vi "newDDreference.vi"(0 "Engine Reference":refnum<k7>, 5 "Sequence File Ref":refnum<k7>, 11 "error in":errorcluster) -> (4 "Engine Reference (out)":refnum<k7>, 6 "Sequence File (out)":refnum<k7>, 15 "error out":errorcluster)   [LabVIEW 2010]
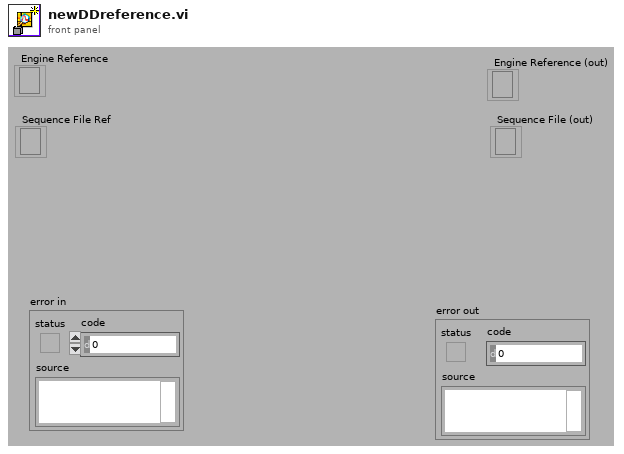
[diagram p1: front panel]
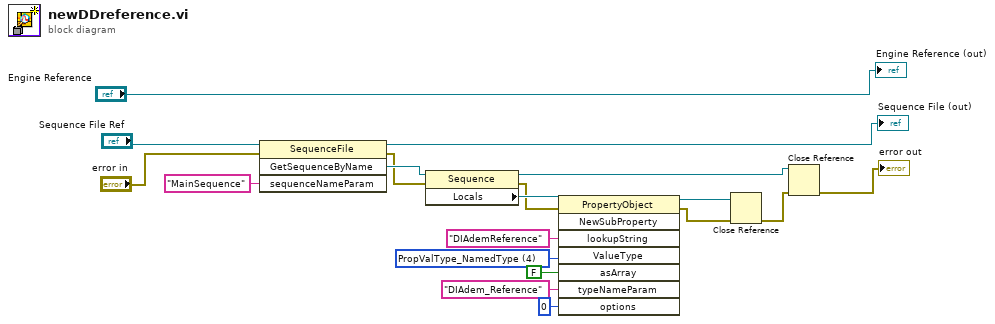
[diagram p0: block diagram]
diagram:
  w15 = 4 items=["PropValType_Container", "PropValType_String", "PropValType_Boolean", "PropValType_Number", "PropValType_NamedType", "PropValType_Reference", "PropValType_Array"] ("ValueType")
  n1 = invoke class="SequenceFile" method="GetSequenceByName"(reference="Sequence File Ref", error in="error in", "sequenceNameParam"="MainSequence") -> (reference out=→"Sequence File (out)":refnum<k7>, error out=w1:errorcluster, "GetSequenceByName"=w18:refnum<k7>)  [unwired: 1 in, 1 out]
  n2 = property class="Sequence"(reference=w18, error in=w1) -> (reference out=w7:refnum<k7>, error out=w9:errorcluster, "Locals"=w17:refnum<k7>)
  n3 = invoke class="PropertyObject" method="NewSubProperty"(reference=w17, error in=w9, "lookupString"="DIAdemReference", "ValueType"=w15, "asArray"=FALSE, "typeNameParam"="DIAdem_Reference", "options"=0) -> (reference out=w11:refnum<k7>, error out=w10:errorcluster)  [unwired: 1 in, 6 out]
  n4 = Close Reference(reference=w11, error in (no error)=w10) -> (error out=w8:errorcluster)
  n5 = Close Reference(reference=w7, error in (no error)=w8) -> (error out=→"error out":errorcluster)
  "Engine Reference (out)" <- "Engine Reference"
